vi "VCS Open Device.vi"(8 "error in (no error)":errorcluster, 11 "device in":T1={"deviceName"="EPOS2", "protocolStackName"="MAXON SERIAL V2", "interfaceName"="USB", "portName"="USB0"}) -> (0 "error out":errorcluster, 3 "keyHandle out":u32)   [LabVIEW 2019, in "maxonEPOS.lvlib"]
doc: "<B>VCS Open Device</B> opens the port for sending and receiving commands."
uses:
  Examples/maxonEPOS.lvlib
  Resources/EposCmd.dll
  Resources/EposCmd64.dll
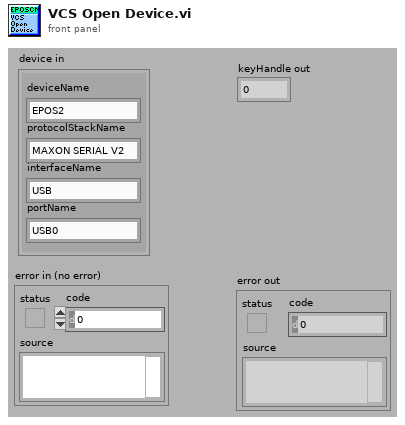
[diagram p1: front panel]
types:
  T1 = cluster{"deviceName":string, "protocolStackName":string, "interfaceName":string, "portName":string}
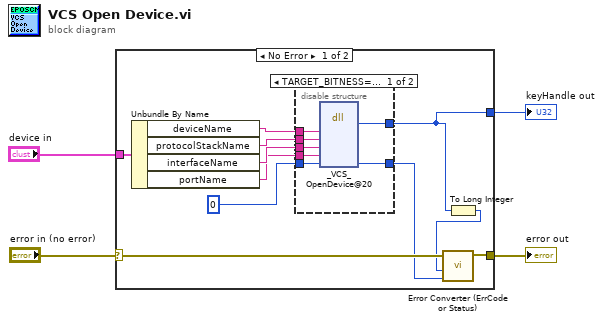
[diagram p0: block diagram]
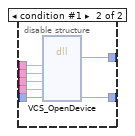
[diagram p2: hidden frame]
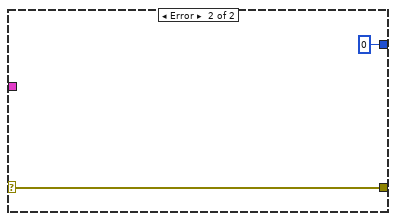
[diagram p3: hidden frame]
diagram:
  n1 = case shown="No Error" "error in (no error)" {
    selector: "error in (no error)" -> [w15 w31]
    tunnel: [w14 w31] -> w3
    tunnel: "device in" -> [w12 _]
    tunnel: [w6 u32 0] -> w1
    frame No Error {
      n2 = Unbundle By Name(w12) -> ("deviceName"=w11:string, "protocolStackName"=w10:string, "interfaceName"=w9:string, "portName"=w8:string)
      n3 = disable-structure shown="TARGET_BITNESS==32, Standard" {
        disable-tunnel: [w22 w29] -> w13
        disable-tunnel: w11 -> [w21 w28]
        disable-tunnel: w10 -> [w20 w27]
        disable-tunnel: w9 -> [w19 w26]
        disable-tunnel: w8 -> [w18 w25]
        disable-tunnel: u32 0 ("pErrorCode") -> [w17 w24]
        disable-tunnel: [w16 w23] -> w6
        frame condition #0 (active) {
          n4 = dll-call lib="C:/workspace/project/scancon/sw/SSI_Tool/InstrumentsInterfaces/Motordriver/maxon EPOS/Resources/EposCmd.dll" fn="_VCS_OpenDevice@20"("DeviceName"=w21, "ProtocolStackName"=w20, "InterfaceName"=w19, "PortName"=w18, "pErrorCode"=w17) -> (w16:u32, "pErrorCode"=w22:u32)  [unwired: 7 in, 2 out]
        }
        frame condition #1 {
          n5 = dll-call lib="C:/Sources/LabView/maxon EPOS/Resources/EposCmd64.dll" fn="VCS_OpenDevice"("DeviceName"=w28, "ProtocolStackName"=w27, "InterfaceName"=w26, "PortName"=w25, "pErrorCode"=w24) -> ("return type"=w23:u32, "pErrorCode"=w29:u32)  [unwired: 7 in, 2 out]
        }
      }
      n6 = To Long Integer(number=w6) -> (32bit integer=w5:i32)
      n7 = call "Error Converter (ErrCode or Status).vi"("error code"=w13, "return type"=w5, "error in (no error)"=w15) -> ("error out"=w14:errorcluster)  [unwired: 7 in]
    }
    frame Error {
    }
  }
  "error out" <- w3
  "keyHandle out" <- w1
